vi "AK Tester manuell.vi"() -> ()   [LabVIEW 2020, in "AK-Schnittstelle.lvlib"]
uses:
  AK-Schnittstelle.lvlib
  AK TCP/AK TCP.lvlib
panel:
  out "Daten (Ausgang) 2":string
  out "Array 2":string[](array[string])
  out "Teil-String":string
  out "Verknüpfter String":string
  out "Array":string[](array[string])
  out "Daten (Ausgang)":string
  in  "String":string
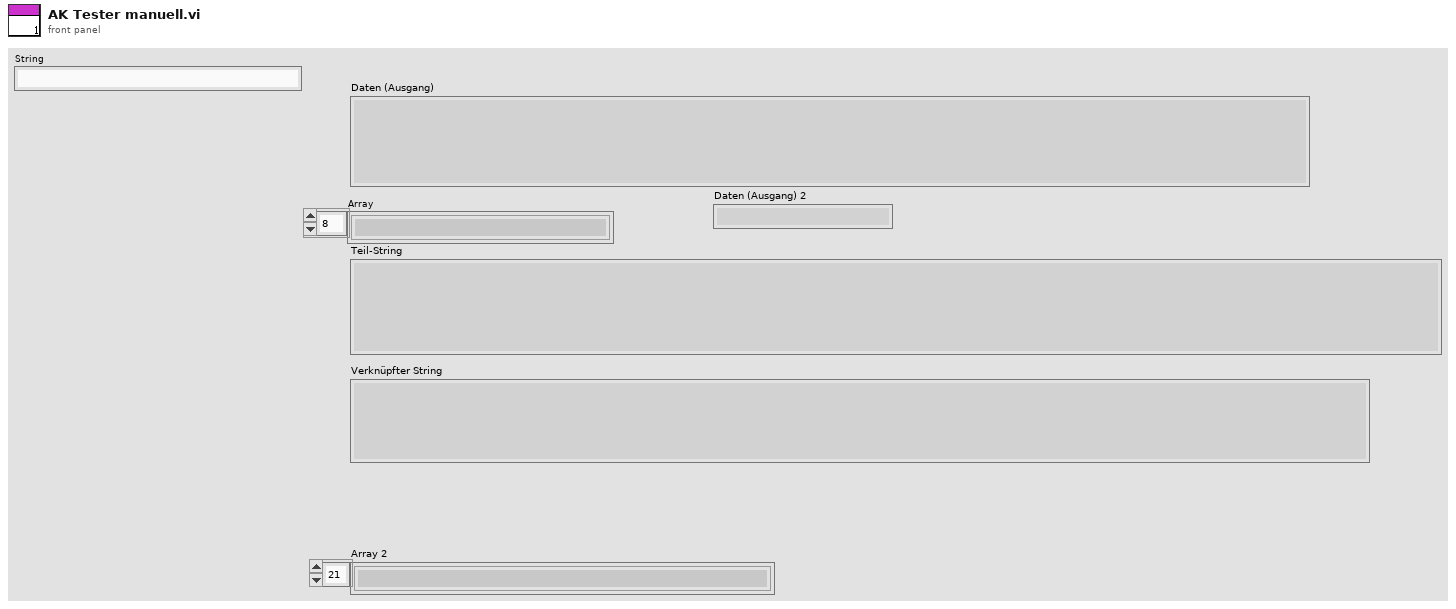
[diagram p1: front panel]
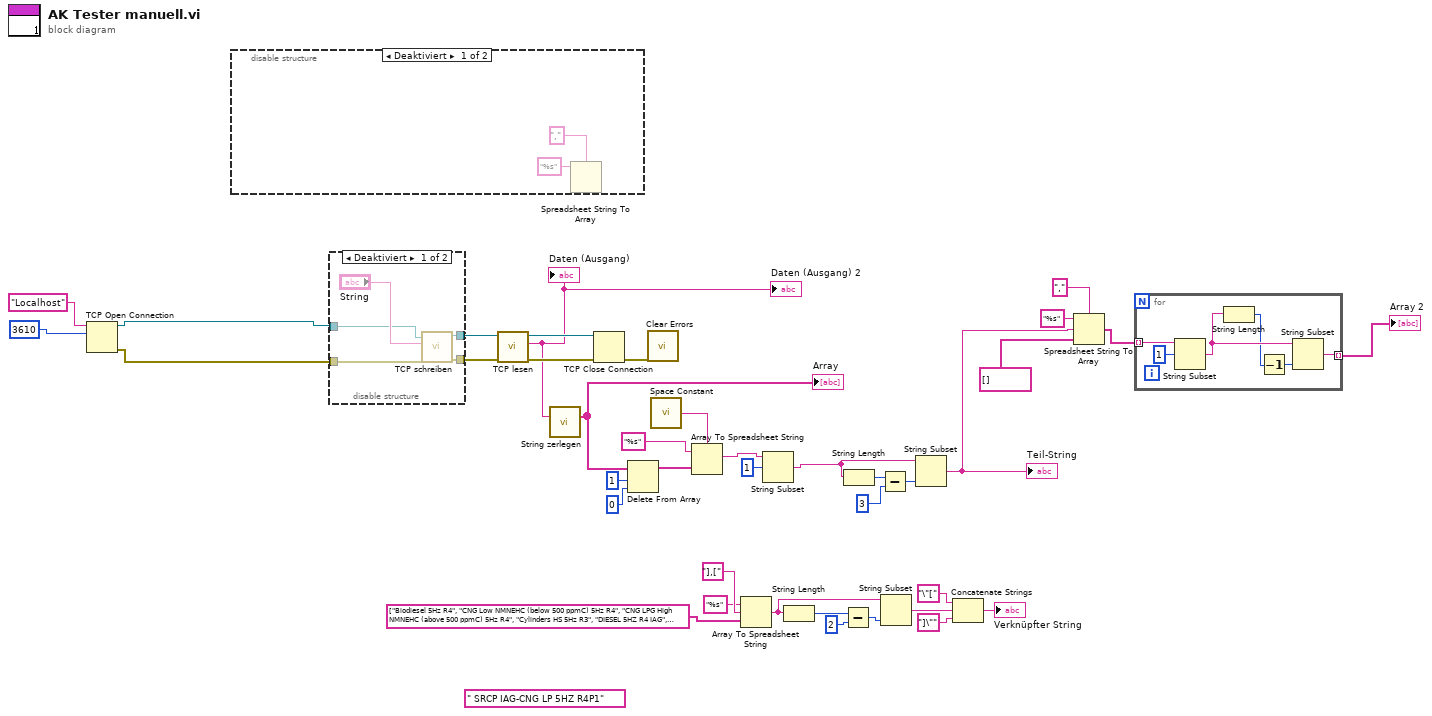
[diagram p0: block diagram]
diagram:
  (unwired) " SRCP IAG-CNG LP 5HZ R4P1"
  n1 = TCP Open Connection(address="Localhost" ("Adresse"), remote port or service name=u16 3610 ("Netzwerk-Port oder -Dienst")) -> (connection ID=w37:refnum<k5>, error out=w38:errorcluster)  [unwired: 3 in]
  n2 = disable-structure shown="Deaktiviert" {
    frame Disabled {
      n3 = Spreadsheet String To Array(delimiter (Tab)="," ("Trennzeichen (Tabulator)"), format string="%s" ("Format-String")) -> ()  [unwired: 2 in, 1 out]
    }
    frame Enabled {
    }
  }
  n4 = disable-structure shown="Deaktiviert" {
    disable-tunnel: [w45 _] -> w35
    disable-tunnel: [w44 _] -> w34
    disable-tunnel: w38 -> [w43 _]
    disable-tunnel: w37 -> [w42 _]
    frame Disabled {
      n5 = call "TCP schreiben.vi"("error in"=w43, "String"="String", "connection ID"=w42) -> ("error out"=w44:errorcluster, "connection ID"=w45:refnum<k5>)  [unwired: 6 in, 1 out]
    }
    frame Enabled {
    }
  }
  n6 = call "TCP lesen.vi"("Fehler (Eingang)"=w34, "connection ID"=w35) -> ("error out"=w32:errorcluster, "Daten (Ausgang)"=w13:string, "connection ID"=w33:refnum<k5>)  [unwired: 7 in]
  "Daten (Ausgang)" <- w13
  "Daten (Ausgang) 2" <- w13
  n7 = call "String zerlegen.vi"("read buffer"=w13) -> ("Array"=w20:string[])  [unwired: 14 in]
  "Array" <- w20
  n8 = TCP Close Connection(connection ID=w33, error in (no error)=w32) -> (error out=w31:errorcluster)  [unwired: 1 in, 1 out]
  n9 = Delete From Array(array=w20, length=1 ("Länge"), index=0 ("Index")) -> (array with subset deleted=w14:string[])  [unwired: 1 out]
  n10 = call <vilib>:"Clear Errors.vi"("error in (no error)"=w31) -> ()  [unwired: 5 in, 2 out]
  n11 = call <vilib>:"Space Constant.vi"() -> ("String"=w18:string)
  n12 = Array To Spreadsheet String(delimiter (Tab)=w18, array=w14, 3:"%s" ("Format-String")) -> (spreadsheet string=w1:string)
  n13 = Array To Spreadsheet String(delimiter (Tab)="],[" ("Trennzeichen (Tabulator)"), array=string[] ["Biodiesel 5Hz R4", "CNG Low NMNEHC (below 500 ppmC) 5Hz R4", "CNG LPG High NMNEHC (above 500 ppmC) 5Hz R4", "Cylinders HS 5Hz R3", "DIESEL 5HZ R4 IAG", "Diesel 5Hz R4", "Diesel Extended 5Hz R4", "Diesel HS 5Hz R3", "DME 5Hz R4", "Dual Fuel Diesel CNG 5Hz R4", "E5-E85 5Hz R4", "Ethanol 5Hz R4", "Ethanol HS 5Hz R3", "Gasoline 5Hz R4", "Gasoline-E85 HS 5Hz R3", "IAG-CNG LP 5HZ R4P1", "IAG-CNG LP 5Hz SM R4p1", "IAG-DIESEL LP 5HZ R4p1", "IAG-DIESEL LP 5HZ SM R4p1", "IAG-GASOLINE LP 5HZ R4P1", "IAG-GASOLINE LP 5Hz SM R4p1", "NG Engines HS 5Hz R3"] ("Array 2"), 3:"%s" ("Format-String")) -> (spreadsheet string=w3:string)
  n14 = String Subset(string=w1, offset (0)=1 ("Offset (0)")) -> (substring=w12:string)  [unwired: 1 in]
  n15 = String Length(string=w3) -> (length=w25:i32)
  n16 = Subtract(x=w25, y=2) -> (x-y=w23:i32)
  n17 = String Length(string=w12) -> (length=w15:i32)
  n18 = Subtract(x=w15, y=3) -> (x-y=w17:i32)
  n19 = String Subset(string=w3, length (rest)=w23) -> (substring=w27:string)  [unwired: 1 in]
  n20 = String Subset(string=w12, length (rest)=w17) -> (substring=w6:string)  [unwired: 1 in]
  "Teil-String" <- w6
  n21 = Concatenate Strings("\"[" ("String"), w27, "]\"") -> (→"Verknüpfter String":string)
  n22 = Spreadsheet String To Array(delimiter (Tab)="," ("Trennzeichen (Tabulator)"), format string="%s" ("Format-String"), spreadsheet string=w6, array type (2D Dbl)=string[] []) -> (array=w7:string[])
  n23 = for {
    tunnel: w7 -> [w52] mode=indexing
    tunnel: [w47] -> w5 mode=indexing
    n24 = String Subset(string=w52, offset (0)=1 ("Offset (0)")) -> (substring=w50:string)  [unwired: 1 in]
    n25 = String Length(string=w50) -> (length=w48:i32)
    n26 = Decrement(x=w48) -> (x-1=w49:i32)
    n27 = String Subset(string=w50, length (rest)=w49) -> (substring=w47:string)  [unwired: 1 in]
  }
  "Array 2" <- w5
